vi "ReadI16FITS.vi"(3 "error in":errorcluster, 4 "Plane# (0..NAXIS3-1)":u16, 5 "file path":path) -> (0 "error out":errorcluster, 2 "u16 pixmap":u16[][](array[numeric]))   [LabVIEW 2011]
panel:
  out "Intensity Graph":u16[][](graph)
  out "FITS":T1
  # "this is IJ-Orientation"
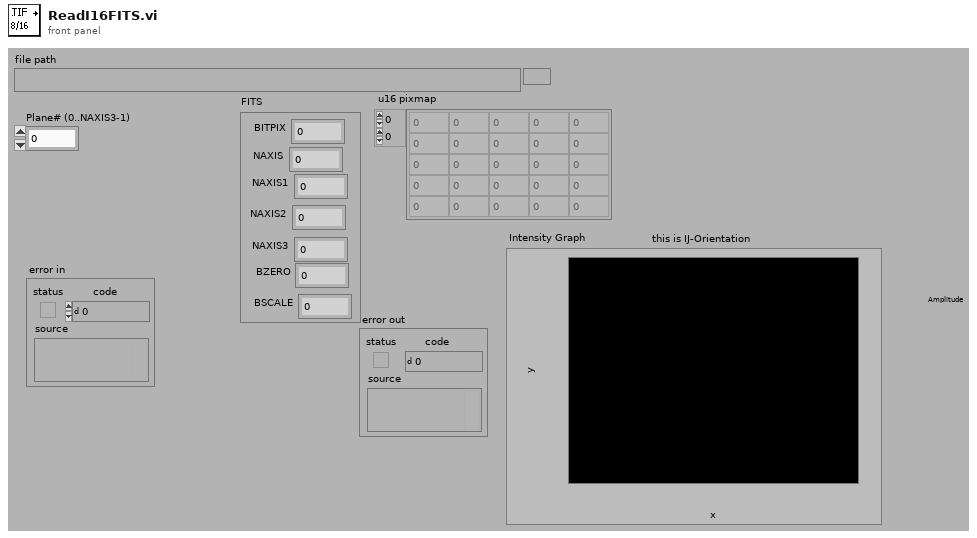
[diagram p1: front panel]
types:
  T1 = cluster{"BITPIX":i16, "NAXIS":i16, "NAXIS1":u16, "NAXIS2":u16, "NAXIS3":u16, "BZERO":dbl, "BSCALE":dbl}
  T2 = cluster{"fits refnum":refnum<file>, "Byte-Reihenfolge (0:Big-Endian, 2:LSB)":enum16{"big-endian, network order", "native, host order", "little-endian"}}
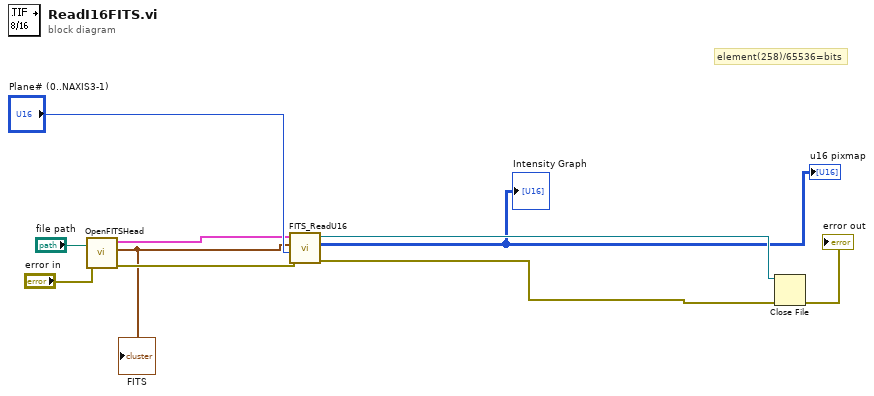
[diagram p0: block diagram]
diagram:
  # "element(258)/65536=bits"
  n1 = call "OpenFITSHead.vi"("file path"="file path", "error in"="error in") -> ("FITS file"=w3:T2, "FITS"=w2:T1, "error out"=w7:errorcluster)  [unwired: 1 in]
  "FITS" <- w2
  n2 = call "FITS_ReadU16.vi"("error in (no error)"=w7, "Plane# (0..n-1)"="Plane# (0..NAXIS3-1)", "FITS"=w2, "FITS file"=w3) -> ("error out"=w6:errorcluster, "Array"=→"u16 pixmap" →"Intensity Graph":u16[][], "Byte Stream File out"=w5:refnum<file>)  [unwired: 5 in]
  n3 = Close File(refnum=w5, error in=w6) -> (error out=→"error out":errorcluster)  [unwired: 1 out]
